vi "DAQ_Digital Clk Gen Close.vi"(0 "DAQmx Task In":refnum<k21>, 11 "error in":errorcluster) -> (15 "error out":errorcluster)   [LabVIEW 2021, in "DAQ_Digital Clock Generation.lvlib"]
doc: "Aborts and clears the Digital Clock Generation task"
uses:
  DAQ_Digital Clock Generation.lvlib
panel:
  # "Inputs"
  # "Outputs"
  # "Overview:\nThis VI closes the digitial clock generation DAQmx Task.\n\nHardware Requirement: A compatible PXI, PCIe, USB, cDAQ or Testscale device\n\nSoftware Requirement: NI DAQmx 2022Q4 or later\n\n\nInstructions:\n1. Input the digitial clock generation task through DAQmx Task In control.\n2. This VI aborts and clears the digitial clock generation task."
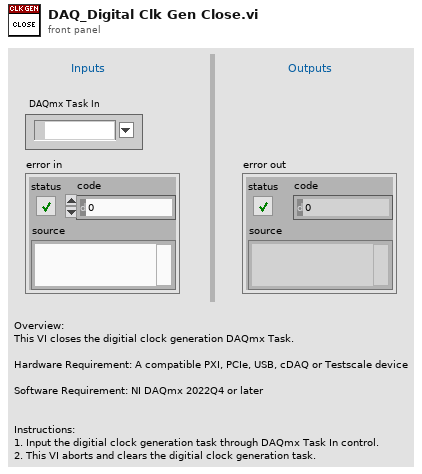
[diagram p1: front panel]
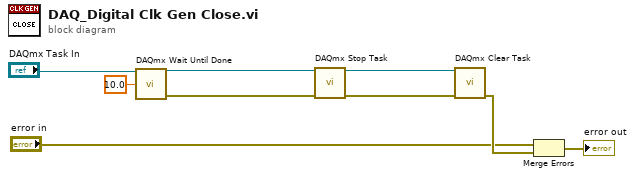
[diagram p0: block diagram]
diagram:
  n1 = call <vilib>:"DAQmx Wait Until Done.vi"("task/channels in"="DAQmx Task In", "timeout (sec)"=10.0) -> ("task out"=w3:refnum<k21>, "error out"=w2:errorcluster)  [unwired: 12 in]
  n2 = call <vilib>:"DAQmx Stop Task.vi"("task/channels in"=w3, "error in"=w2) -> ("task out"=w9:refnum<k21>, "error out"=w8:errorcluster)  [unwired: 12 in]
  n3 = call <vilib>:"DAQmx Clear Task.vi"("task in"=w9, "error in"=w8) -> ("error out"=w6:errorcluster)  [unwired: 13 in]
  n4 = Merge Errors("error in", w6) -> (→"error out":errorcluster)
